vi "read.vi"(8 "error in (no error)":errorcluster, 11 "DigitalSimHardware in":refnum<class "DigitalSimHardware.lvclass">) -> (0 "error out":errorcluster, 2 "outputs":u16[][](array[numeric]), 3 "DigitalSimHardware out":refnum<class "DigitalSimHardware.lvclass">)   [LabVIEW 2017, in "DigitalSimHardware.lvclass"]
doc: "Read data from the instrument"
uses:
  DigitalSimHardware.lvclass
  support/my_global.vi
panel:
  # "2D array of booleans"
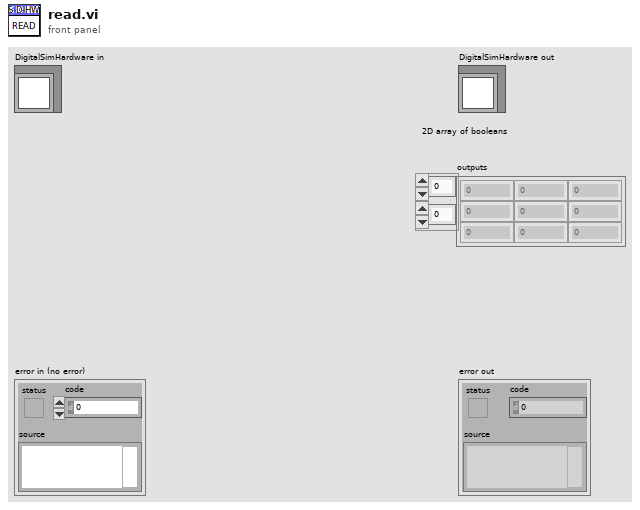
[diagram p1: front panel]
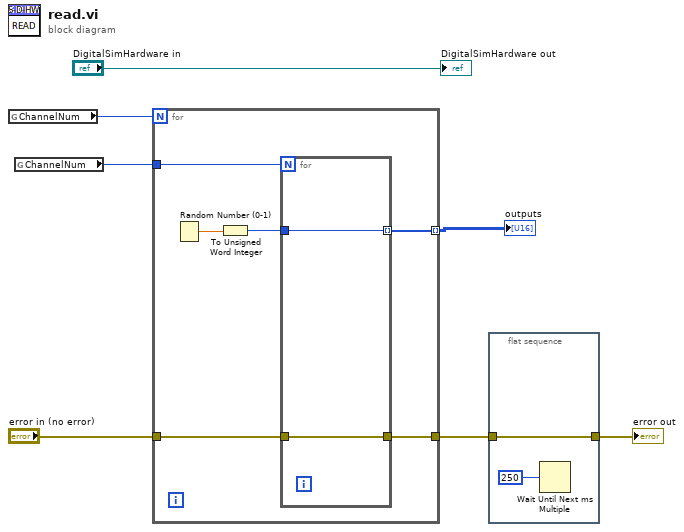
[diagram p0: block diagram]
diagram:
  n1 = global read "my_global.vi" "ChannelNum"() -> (w6:u32)
  n2 = global read "my_global.vi" "ChannelNum"() -> (w4:u32)
  n3 = for {
    N: w6 -> [_]
    tunnel: [w13] -> w5 mode=indexing
    tunnel: w4 -> [w12]
    tunnel: "error in (no error)" -> [w11]
    tunnel: [w10] -> w2
    n4 = Random Number (0-1)() -> (number: 0 to 1=w9:dbl)
    n5 = To Unsigned Word Integer(number=w9) -> (unsigned 16bit integer=w8:u16)
    n6 = for {
      N: w12 -> [_]
      tunnel: [w14] -> w13 mode=indexing
      tunnel: w11 -> [w15]
      tunnel: [w15] -> w10
      tunnel: w8 -> [w14]
    }
  }
  "outputs" <- w5
  n7 = flat-sequence {
    tunnel: w2 -> [w17]
    tunnel: [w17] -> w1
    frame #0 {
      n8 = Wait Until Next ms Multiple(millisecond multiple=u32 250) -> ()  [unwired: 1 out]
    }
  }
  "error out" <- w1
  "DigitalSimHardware out" <- "DigitalSimHardware in"
